vi "SortEigsDescending.vi"(11 "Array in":dbl[](array[numeric])) -> (3 "Array out":dbl[][](array[numeric]))   [LabVIEW 2022 SP3]
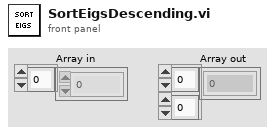
[diagram p1: front panel]
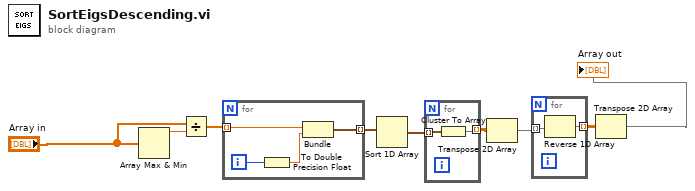
[diagram p0: block diagram]
diagram:
  n1 = Array Max & Min(array="Array in") -> (max value=w2:dbl)  [unwired: 3 out]
  n2 = Divide(x="Array in", y=w2) -> (x/y=w1:dbl[])
  n3 = for {
    tunnel: w1 -> [w13] mode=indexing
    tunnel: [w10] -> w4 mode=indexing
    i -> [w12]
    n4 = To Double Precision Float(number=w12) -> (double precision float=w11:dbl)
    n5 = Bundle(w13, w11) -> (w10:cluster{dbl, dbl})  [unwired: 1 in]
  }
  n6 = Sort 1D Array(array=w4) -> (sorted array=w3:cluster{dbl, dbl}[])
  n7 = for {
    tunnel: w3 -> [w15] mode=indexing
    tunnel: [w14] -> w5 mode=indexing
    n8 = Cluster To Array(cluster=w15) -> (array=w14:dbl[])
  }
  n9 = Transpose 2D Array(2D array=w5) -> (transposed array=w6:dbl[][])
  n10 = for {
    tunnel: w6 -> [w17] mode=indexing
    tunnel: [w16] -> w7 mode=indexing
    n11 = Reverse 1D Array(array=w17) -> (reversed array=w16:dbl[])
  }
  n12 = Transpose 2D Array(2D array=w7) -> (transposed array=→"Array out":dbl[][])
